vi "LvIRKit_InputButtonName_Panel.vi"(11 "button name":string) -> (1 "buttunName":string, 2 "Cancel?":bool)   [LabVIEW 2014]
panel:
  in  "Button":string(combo)="電源" caption="ボタン"
  in  "Type":string(combo)="TV" caption="機器"
  in  "Place":string(combo)="リビング" caption="場所"
  out "name":string caption="登録名"
  in  "Btn Cancel":bool
  in  "Btn OK":bool
  # "ボタンの名前を入力してください"
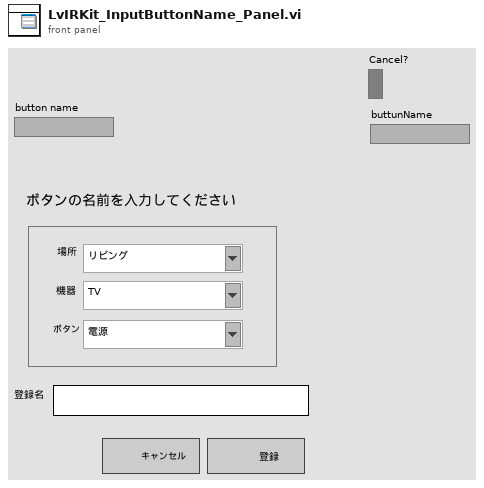
[diagram p1: front panel]
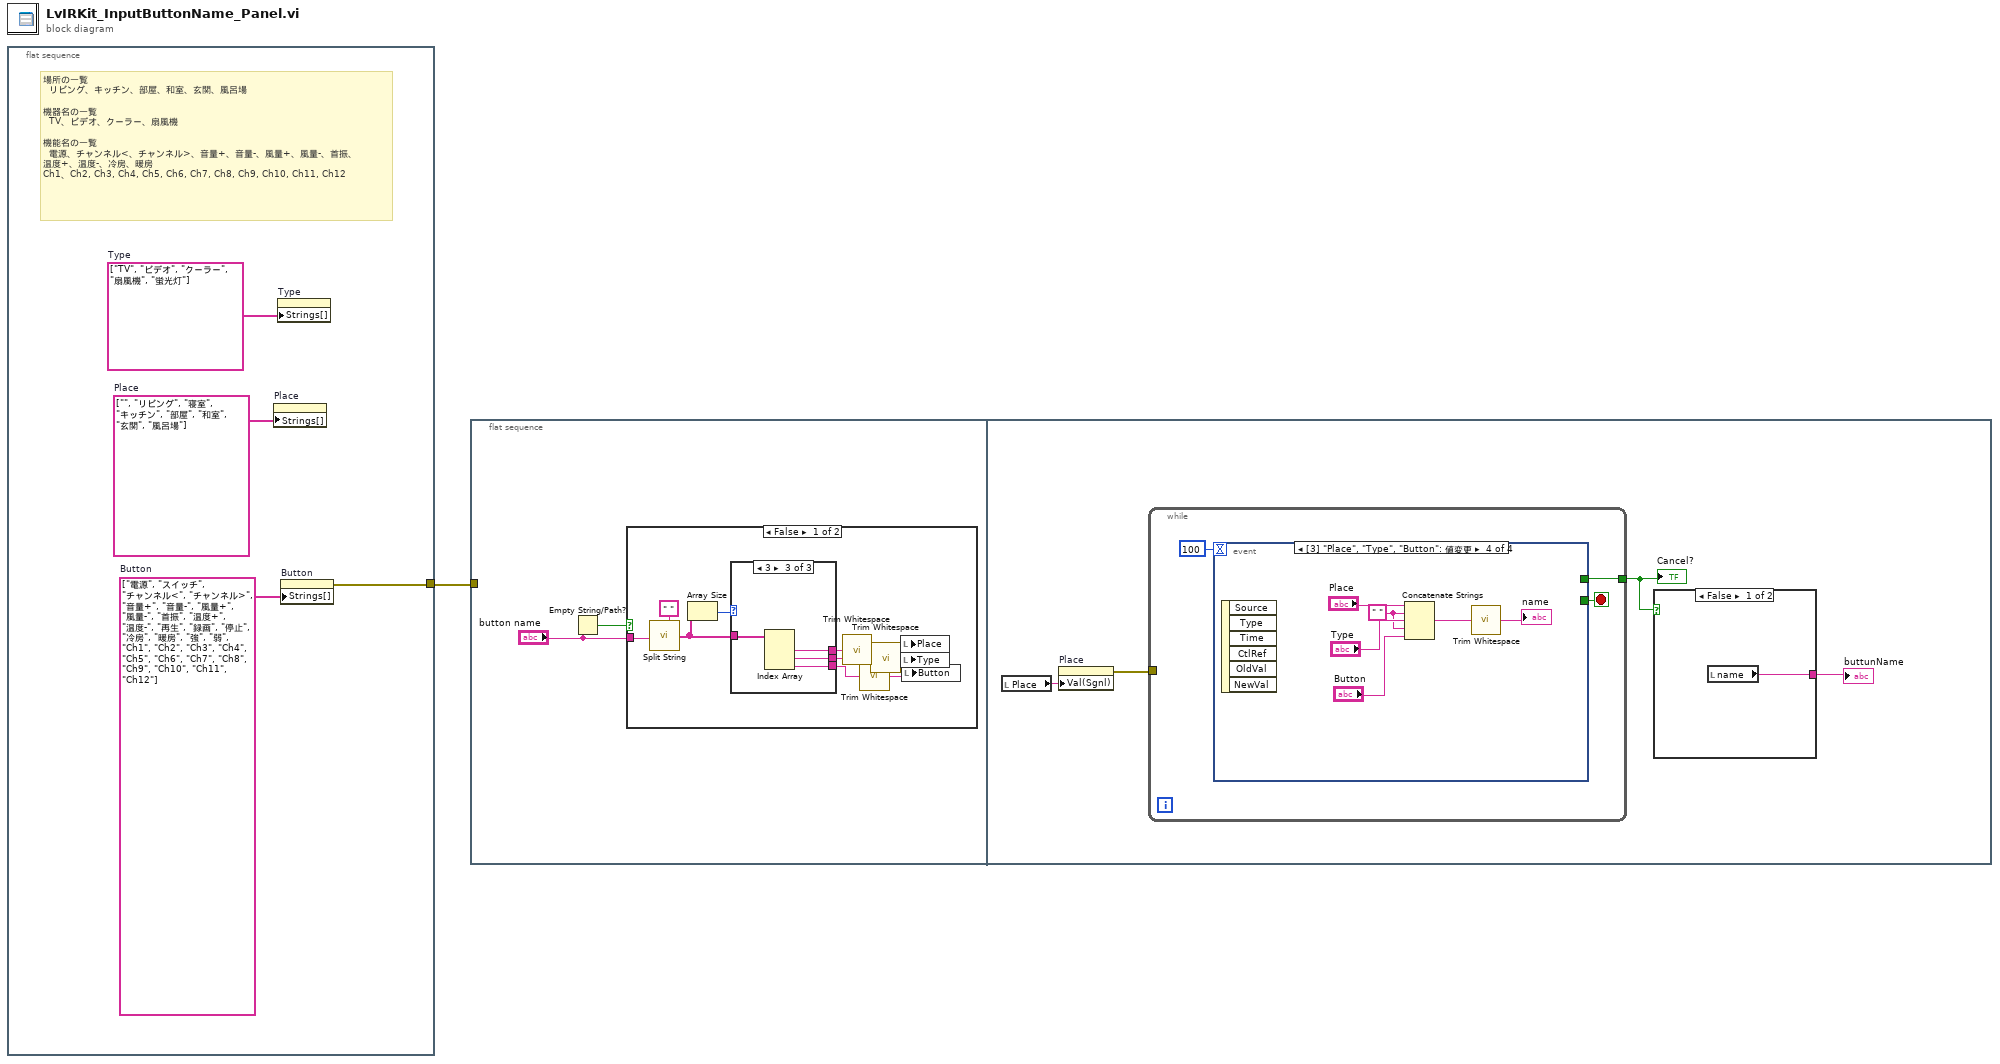
[diagram p0: block diagram]
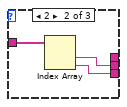
[diagram p3: hidden frame]
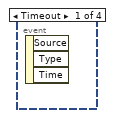
[diagram p6: hidden frame]
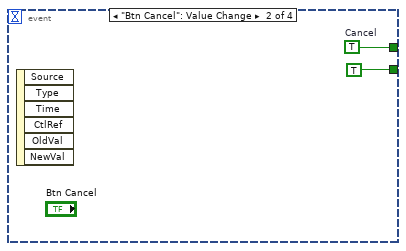
[diagram p7: hidden frame]
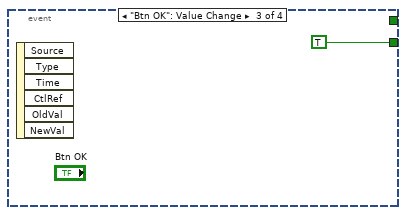
[diagram p8: hidden frame]
diagram:
  n1 = flat-sequence {
    tunnel: [w2] -> w1
    frame #0 {
      w3 = string[] ["電源", "スイッチ", "チャンネル<", "チャンネル>", "音量+", "音量-", "風量+", "風量-", "首振", "温度+", "温度-", "再生", "録画", "停止", "冷房", "暖房", "強", "弱", "Ch1", "Ch2", "Ch3", "Ch4", "Ch5", "Ch6", "Ch7", "Ch8", "Ch9", "Ch10", "Ch11", "Ch12"]  # Button
      w4 = string[] ["", "リビング", "寝室", "キッチン", "部屋", "和室", "玄関", "風呂場"]  # Place
      w5 = string[] ["TV", "ビデオ", "クーラー", "扇風機", "蛍光灯"]  # Type
      # "場所の一覧\n  リビング、キッチン、部屋、和室、玄関、風呂場\n\n機器名の一覧\n  TV、ビデオ、クーラー、扇風機\n\n機能名の一覧\n  電源、チャンネル<、チャンネル>、音量+、音量-、風量+、風量-、首振、\n温度+、温度-、冷房、暖房\nCh1、Ch2, Ch3, Ch4, Ch5, Ch6, Ch7, Ch8, Ch9, Ch10, Ch11, Ch12"
      n2 = property on="Place" class="CmbBox"("Strings[]"=w4) -> ()  [unwired: 2 in, 2 out]
      n3 = property on="Type" class="CmbBox"("Strings[]"=w5) -> ()  [unwired: 2 in, 2 out]
      n4 = property on="Button" class="CmbBox"("Strings[]"=w3) -> (error out=w2:errorcluster)  [unwired: 2 in, 1 out]
    }
  }
  n5 = flat-sequence {
    tunnel: w1 -> [_]
    frame #0 {
      n6 = Empty String/Path?(string/path="button name") -> (empty?=w7:bool)
      n7 = case shown="FALSE" w7 {
        tunnel: "button name" -> [w17 _]
        frame False {
          n8 = call <vilib>:"Split String.vi"("Split Pattern"=" ", "Input String"=w17) -> ("Split String"=w14:string[])  [unwired: 5 in]
          n9 = Array Size(array=w14) -> (size(s)=w15:i32)
          n10 = case shown="3" w15 {
            tunnel: w14 -> [_ w20 w24]
            tunnel: [_ _ w23] -> w13
            tunnel: [_ w19 w22] -> w12
            tunnel: [_ w18 w21] -> w11
            frame Default {
            }
            frame 2 {
              n11 = Index Array(array=w20) -> (element #1=w19:string, element #2=w18:string)  [unwired: 2 in]
            }
            frame 3 {
              n12 = Index Array(array=w24) -> (element #1=w23:string, element #2=w22:string, element #3=w21:string)  [unwired: 3 in]
            }
          }
          n13 = call <vilib>:"Trim Whitespace.vi"("string"=w13) -> ("trimmed string"=w10:string)  [unwired: 1 in]
          n14 = call <vilib>:"Trim Whitespace.vi"("string"=w11) -> ("trimmed string"=w8:string)  [unwired: 1 in]
          n15 = call <vilib>:"Trim Whitespace.vi"("string"=w12) -> ("trimmed string"=w9:string)  [unwired: 1 in]
          n16 = local write "Place"(w10) -> ()
          n17 = local write "Type"(w9) -> ()
          n18 = local write "Button"(w8) -> ()
        }
        frame True {
        }
      }
    }
    frame #1 {
      n19 = local read "Place"() -> (w28:string)
      n20 = property on="Place" class="CmbBox"("Val(Sgnl)"=w28) -> (error out=w27:errorcluster)  [unwired: 2 in, 1 out]
      n21 = while {
        tunnel: w27 -> [_]
        tunnel: [w30] -> w25
        stop <- w31 stop-if-true
        n22 = event shown="[3] \"Place\", \"Type\", \"Button\": 値変更" {
          selector: _ -> [_ _ _ _]
          dyn-events: _ -> [_ _ _ _]
          timeout: 100 -> [_ _ _ _]
          tunnel: [_ TRUE TRUE _] -> w31
          tunnel: [_ w33 _ _] -> w30
          event Timeout {
            n23 = event-data() -> ()  [unwired: 1 in, 3 out]
          }
          event "Btn Cancel": Value Change {
            w33 = TRUE  # Cancel
            n24 = event-data() -> ()  [unwired: 1 in, 6 out]
          }
          event "Btn OK": Value Change {
            n25 = event-data() -> ()  [unwired: 1 in, 6 out]
          }
          event "Place", "Type", "Button": Value Change {
            w37 = " " ("文字列")
            n26 = event-data() -> ()  [unwired: 1 in, 6 out]
            n27 = Concatenate Strings("Place", w37, "Type", w37, "Button") -> (w41:string)
            n28 = call <vilib>:"Trim Whitespace.vi"("string"=w41) -> ("trimmed string"=→"name":string)  [unwired: 1 in]
          }
        }
      }
      "Cancel?" <- w25
      n29 = case shown="FALSE" w25 {
        tunnel: [w29 _] -> w26
        frame False {
          n30 = local read "name"() -> (w29:string)
        }
        frame True {
        }
      }
      "buttunName" <- w26
    }
  }
